vi "_test_formattingJUnitFromResult__2.vi"() -> ()   [LabVIEW 2020, in "Caraya.lvlib" / "Test Report.JUnit.lvclass"]
uses:
  Test Report.JUnit.lvclass
  MsgSerializer.XML/MsgSerializer.XML.lvclass
  MsgSerializer.XML/format -- enum.ctl
  Test Result/Node Results (Extended).ctl
  Test Result/Test Node (Extended).ctl
  Test Result/Test Registration Data.ctl
  Test Result/Assert Event Data (Extended).ctl
  MsgSerializer.XML/MsgSerializer.XML.lvclass/MsgSerializer.XML.ctl
  Test Result/Test Result.lvclass
panel:
  out "Array 2":string[](array[string])
  out "Array":string[](array[string])
  out "Serialized Message":string
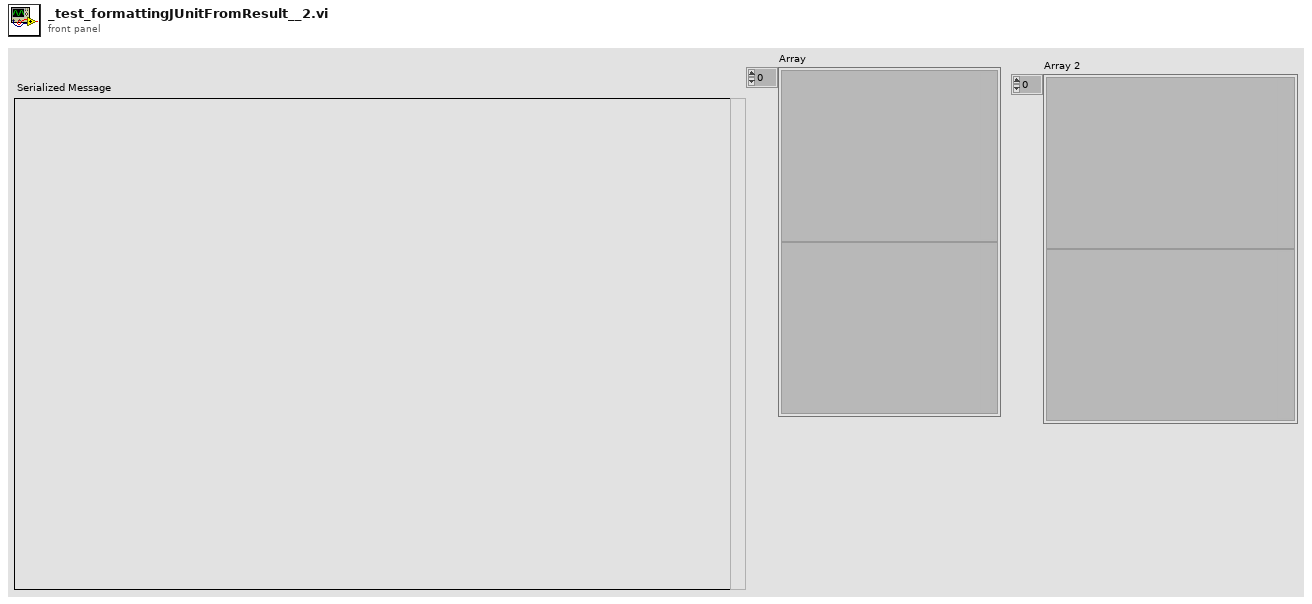
[diagram p1: front panel]
types:
  T1 = typedef "Caraya.lvlib/Test Result.lvclass/Node Results (Extended).ctl" = cluster{"Test Node":T2, "Assertions":T4[]}
  T2 = typedef "Caraya.lvlib/Test Result.lvclass/Test Node (Extended).ctl" = cluster{"Test Registration":T3, "Defined":bool, "Passed":bool, "properties":variant}
  T3 = typedef "Caraya.lvlib/Test Result.lvclass/Test Registration Data.ctl" = cluster{"Name":string, "Call Chain":string[], "Time Stamp":timestamp, "Test ID":string, "Caller ID":string}
  T4 = typedef "Caraya.lvlib/Test Result.lvclass/Assert Event Data (Extended).ctl" = cluster{"name":string, "passed":bool, "call-chain":string[], "test-error":errorcluster, "timestamp":timestamp, "assert-id":string, "test-id":string, "time":dbl, "message":string, "properties":variant, "measurements":variant, "user-defined":variant}
  T5 = typedef "Caraya.lvlib/MsgSerializer.XML.lvclass/format -- enum.ctl" = enum16{"value", "tag", "property"}
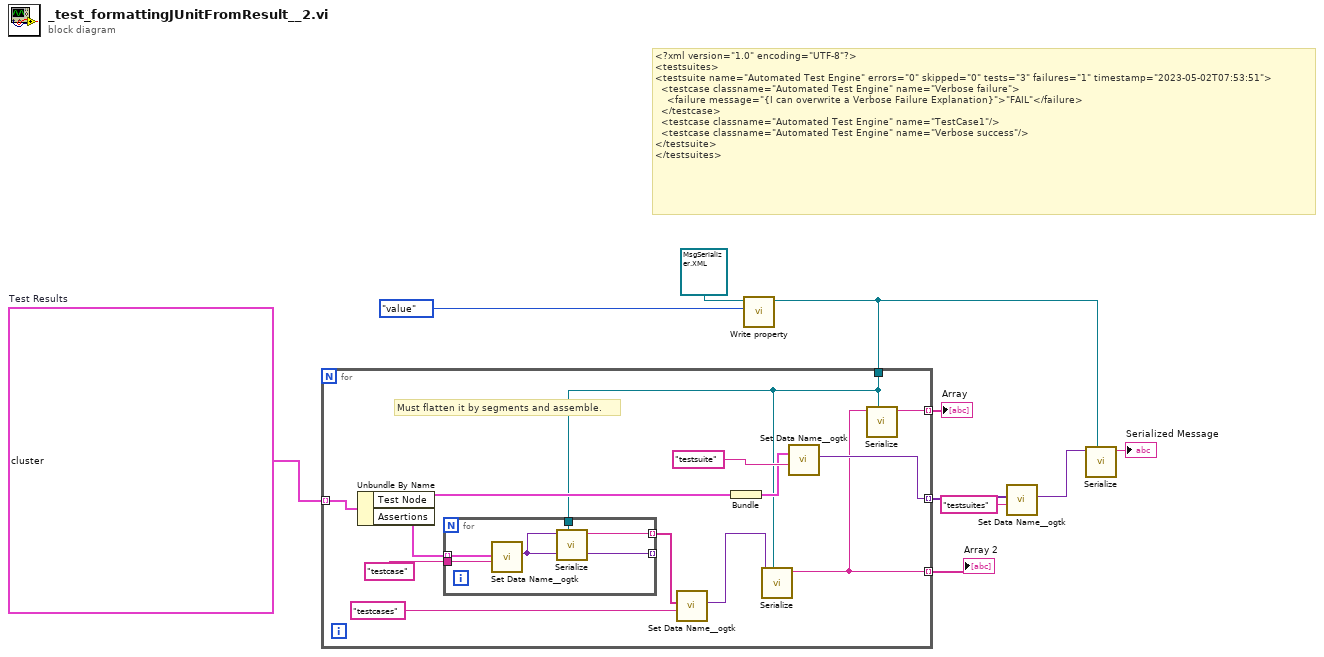
[diagram p0: block diagram]
diagram:
  w8 = T1[] [{"Test Node"={"Test Registration"={"Name"="Test Properties Report (XML).vi", "Call Chain"=[], "Time Stamp"=timestamp(3765884031.4811797 s since 1904-01-01), "Test ID"="Test Properties Report (XML).vi:000001", "Caller ID"=""}, "Defined"=FALSE, "Passed"=FALSE, "properties"=variant}, "Assertions"=[]}, {"Test Node"={"Test Registration"={"Name"="Automated Test Engine", "Call Chain"=["Test Assert Properties.vi", "Test Properties Report (XML).vi"], "Time Stamp"=timestamp(3765884031.4811797 s since 1904-01-01), "Test ID"="Automated Test Engine:000002", "Caller ID"="Test Properties Report (XML).vi:000001"}, "Defined"=TRUE, "Passed"=FALSE, "properties"=variant("hyperlink"=variant(string "https://github.com/JKISoftware/Caraya"), "requirement-id"=variant(string "ID-0001-0001"))}, "Assertions"=[{"name"="Verbose failure", "passed"=FALSE, "call-chain"=["Test Assert Properties.vi", "Test Properties Report (XML).vi"], "test-error"={"status"=FALSE, "code"=0, "source"=""}, "timestamp"=timestamp(3765884031.4811797 s since 1904-01-01), "assert-id"="035648::390030", "test-id"="Automated Test Engine:000002", "time"=-1.0, "message"="I can overwrite a Verbose Failure Explanation", "properties"=variant, "measurements"=variant, "user-defined"=variant}, {"name"="TestCase1", "passed"=TRUE, "call-chain"=["Test Assert Properties.vi", "Test Properties Report (XML).vi"], "test-error"={"status"=FALSE, "code"=0, "source"=""}, "timestamp"=timestamp(3765884031.4811797 s since 1904-01-01), "assert-id"="035649::390045", "test-id"="Automated Test Engine:000002", "time"=-1.0, "message"="", "properties"=variant("description"=variant(string "Minimum Rail Voltage"), "eval"=variant(string "voltage >= 3,200000")), "measurements"=variant("voltage"=variant(dbl 3.3046)), "user-defined"=variant}, {"name"="Verbose success", "passed"=TRUE, "call-chain"=["Test Assert Properties.vi", "Test Properties Report (XML).vi"], "test-error"={"status"=FALSE, "code"=0, "source"=""}, "timestamp"=timestamp(3765884031.483181 s since 1904-01-01), "assert-id"="035650::390030", "test-id"="Automated Test Engine:000002", "time"=-1.0, "message"="I can explain the reason of a successful assertion", "properties"=variant, "measurements"=variant, "user-defined"=variant}]}]  # Test Results
  # "<?xml version=\"1.0\" encoding=\"UTF-8\"?>\n<testsuites>\n<testsuite name=\"Automated Test Engine\" errors=\"0\" skipped=\"0\" tests=\"3\" failures=\"1\" timestamp=\"2023-05-02T07:53:51\">\n  <testcase classname=\"Automated Test Engine\" name=\"Verbose failure\">\n    <failure message=\"{I can overwrite a Verbose Failure Explanation}\">\"FAIL\"</failure>\n  </testcase>\n  <testcase classname=\"Automated Test Engine\" name=\"TestCase1\"/>\n  <testcase classname=\"Automated Test Engine\" name=\"Verbose success\"/>\n</testsuite>\n</testsuites>"
  n1 = call "Write property.vi"("format"=format_--_enum."value", "MsgSerializer.XMLProperty in"=refnum<class "MsgSerializer.XML.lvclass"> refnum ("Caraya.lvlib:MsgSerializer.XML.lvclass")) -> ("MsgSerializer.XMLProperty out"=w3:refnum<class "MsgSerializer.XML.lvclass">)  [unwired: 9 in]
  n2 = for {
    tunnel: w8 -> [w23] mode=indexing
    tunnel: [w16] -> w6 mode=indexing
    tunnel: w3 -> [w13]
    tunnel: [w15] -> w2 mode=indexing
    tunnel: [w14] -> w1 mode=indexing
    # "Must flatten it by segments and assemble."
    n3 = Unbundle By Name(w23) -> ("Test Node"=w20:T2, "Assertions"=w18:T4[])
    n4 = for {
      tunnel: w18 -> [w28] mode=indexing
      tunnel: [w26] -> _ mode=indexing
      tunnel: "testcase" ("Data Name") -> [w27]
      tunnel: w13 -> [w25]
      tunnel: [w24] -> w11 mode=indexing
      n5 = call <userlib>:"Set Data Name__ogtk.vi"("Data Name"=w27, "Data"=w28) -> ("Renamed Data"=w26:variant)  [unwired: 8 in, 1 out]
      n6 = call-dynamic "Serialize.vi"("MsgSerializer"=w25, "Value"=w26) -> ("Serialized Message"=w24:string)  [unwired: 8 in, 1 out]
    }
    n7 = call <userlib>:"Set Data Name__ogtk.vi"("Data Name"="testcases", "Data"=w11) -> ("Renamed Data"=w12:variant)  [unwired: 8 in, 1 out]
    n8 = Bundle("Test Node"=w20) -> (w19:cluster{"Test Node":T2})  [unwired: 1 in]
    n9 = call-dynamic "Serialize.vi"("MsgSerializer"=w13, "Value"=w12) -> ("Serialized Message"=w14:string)  [unwired: 8 in, 1 out]
    n10 = call <userlib>:"Set Data Name__ogtk.vi"("Data Name"="testsuite", "Data"=w19) -> ("Renamed Data"=w16:variant)  [unwired: 8 in, 1 out]
    n11 = call-dynamic "Serialize.vi"("MsgSerializer"=w13, "Value"=w14) -> ("Serialized Message"=w15:string)  [unwired: 8 in, 1 out]
  }
  "Array" <- w2
  "Array 2" <- w1
  n12 = call <userlib>:"Set Data Name__ogtk.vi"("Data Name"="testsuites", "Data"=w6) -> ("Renamed Data"=w5:variant)  [unwired: 8 in, 1 out]
  n13 = call-dynamic "Serialize.vi"("MsgSerializer"=w3, "Value"=w5) -> ("Serialized Message"=→"Serialized Message":string)  [unwired: 8 in, 1 out]
